vi "SetClassQueue.vi"(8 "ErrorIn(No Error)":errorcluster caption="entrée d'erreur (pas d'erreur)", 11 "Tools.lvclass":refnum<class "Tools.lvclass">) -> (0 "sortie d'erreur":errorcluster, 3 "Tools.lvclass Out":refnum<class "Tools.lvclass">)   [LabVIEW 2012, in "Tools.lvclass"]
uses:
  Tools.lvclass
  BaseDevice/BaseDevice.lvclass
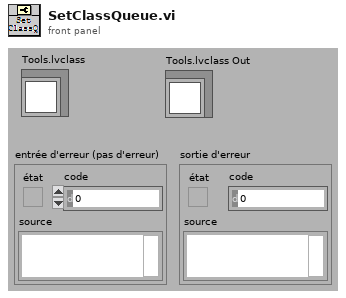
[diagram p1: front panel]
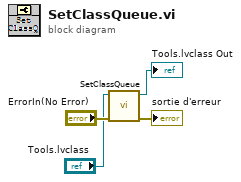
[diagram p0: block diagram]
diagram:
  n1 = call-parent "SetClassQueue.vi"("ErrorIn(No Error)"="ErrorIn(No Error)", "BaseDevice.lvclass"="Tools.lvclass") -> ("sortie d'erreur"=→"sortie d'erreur":errorcluster, "BaseDevice.lvclass Out"=→"Tools.lvclass Out":refnum<class "Tools.lvclass">)  [unwired: 8 in]
